vi "Result_Vectors.vi"(3 "Array":dbl[][](array[numeric])=[[-200.0, -0.1], [-400.0, -0.2], [-600.0, -0.5], [-800.0, -1.0], [-1000.0, -100.0]]) -> (0 "Y-vector":dbl[](array[numeric]), 1 "X-vector":dbl[](array[numeric]))   [LabVIEW 2015]
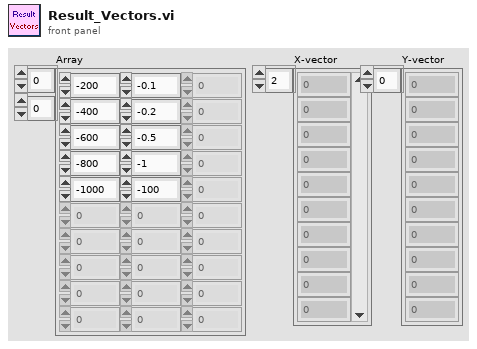
[diagram p1: front panel]
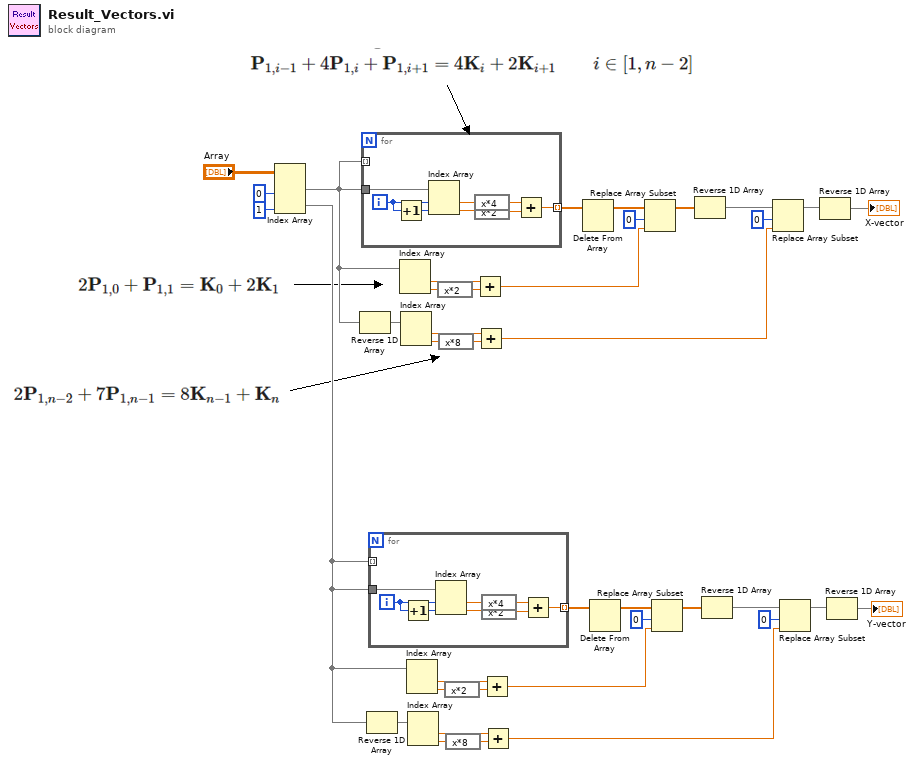
[diagram p0: block diagram]
diagram:
  n1 = Index Array(array="Array", index (col) #1=0 ("disabled index (col)"), index (col) #2=1 ("index (col)")) -> (element #1=w29:dbl[], element #2=w2:dbl[])  [unwired: 2 in]
  n2 = Reverse 1D Array(array=w29) -> (reversed array=w28:dbl[])
  n3 = for {
    tunnel: w29 -> [w47]
    tunnel: w29 -> [_] mode=indexing
    tunnel: [w40] -> w36 mode=indexing
    i -> [w45]
    n4 = Increment(x=w45) -> (x+1=w46:i32)
    n5 = Index Array(array=w47, index #1=w45, index #2=w46) -> (element #1=w44:dbl, element #2=w43:dbl)
    n6 = expression code="x*4"(w44) -> (w42:dbl)
    n7 = expression code="x*2"(w43) -> (w41:dbl)
    n8 = Add(x=w42, y=w41) -> (x+y=w40:dbl)
  }
  n9 = Reverse 1D Array(array=w2) -> (reversed array=w10:dbl[])
  n10 = for {
    tunnel: w2 -> [w55]
    tunnel: w2 -> [_] mode=indexing
    tunnel: [w48] -> w3 mode=indexing
    i -> [w53]
    n11 = Increment(x=w53) -> (x+1=w54:i32)
    n12 = Index Array(array=w55, index #1=w53, index #2=w54) -> (element #1=w52:dbl, element #2=w51:dbl)
    n13 = expression code="x*4"(w52) -> (w50:dbl)
    n14 = expression code="x*2"(w51) -> (w49:dbl)
    n15 = Add(x=w50, y=w49) -> (x+y=w48:dbl)
  }
  n16 = Index Array(array=w29) -> (element #1=w33:dbl, element #2=w35:dbl)  [unwired: 2 in]
  n17 = Index Array(array=w28) -> (element #1=w32:dbl, element #2=w30:dbl)  [unwired: 2 in]
  n18 = Index Array(array=w2) -> (element #1=w6:dbl, element #2=w4:dbl)  [unwired: 2 in]
  n19 = Index Array(array=w10) -> (element #1=w7:dbl, element #2=w9:dbl)  [unwired: 2 in]
  n20 = expression code="x*2"(w35) -> (w34:dbl)
  n21 = expression code="x*8"(w30) -> (w31:dbl)
  n22 = expression code="x*2"(w4) -> (w5:dbl)
  n23 = expression code="x*8"(w9) -> (w8:dbl)
  n24 = Add(x=w33, y=w34) -> (x+y=w25:dbl)
  n25 = Add(x=w32, y=w31) -> (x+y=w21:dbl)
  n26 = Add(x=w6, y=w5) -> (x+y=w13:dbl)
  n27 = Add(x=w7, y=w8) -> (x+y=w17:dbl)
  n28 = Delete From Array(array=w36) -> (array with subset deleted=w27:dbl[])  [unwired: 2 in, 1 out]
  n29 = Delete From Array(array=w3) -> (array with subset deleted=w11:dbl[])  [unwired: 2 in, 1 out]
  n30 = Replace Array Subset(array=w27, new element=w25, index=0) -> (w24:dbl[])
  n31 = Replace Array Subset(array=w11, new element=w13, index=0) -> (w14:dbl[])
  n32 = Reverse 1D Array(array=w24) -> (reversed array=w22:dbl[])
  n33 = Reverse 1D Array(array=w14) -> (reversed array=w16:dbl[])
  n34 = Replace Array Subset(array=w22, new element=w21, index=0) -> (w20:dbl[])
  n35 = Replace Array Subset(array=w16, new element=w17, index=0) -> (w18:dbl[])
  n36 = Reverse 1D Array(array=w20) -> (reversed array=→"X-vector":dbl[])
  n37 = Reverse 1D Array(array=w18) -> (reversed array=→"Y-vector":dbl[])
